vi "均值滤波.vi"(10 "滤波器大小":i32, 11 "inputArray":dbl[][](array[numeric])) -> (1 "中值滤波":dbl[][](array[numeric]), 3 "均值滤波":dbl[][](array[numeric]))   [LabVIEW 2016]
uses:
  <vilib>/Analysis/NI_AALBase.lvlib
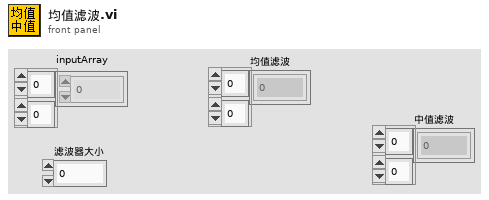
[diagram p1: front panel]
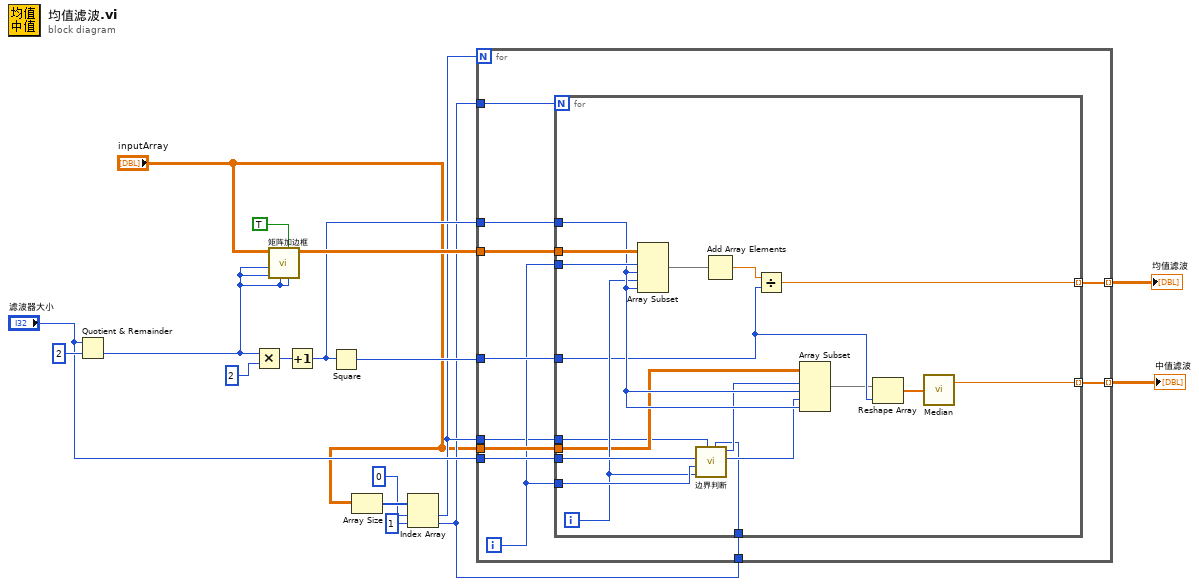
[diagram p0: block diagram]
diagram:
  n1 = Quotient & Remainder(x="滤波器大小", y=2) -> (floor(x/y)=w14:i32)  [unwired: 1 out]
  n2 = Multiply(x=w14, y=2) -> (x*y=w12:i32)
  n3 = call "矩阵加边框.vi"("下边框宽度"=w14, "复制面阵边缘作为边框值"=TRUE, "上边框宽度"=w14, "右边框宽度"=w14, "左边框宽度"=w14, "原面阵"="inputArray") -> ("加边框面阵"=w16:dbl[][])  [unwired: 5 in]
  n4 = Increment(x=w12) -> (x+1=w9:i32)
  n5 = Square(x=w9) -> (x^2=w11:i32)
  n6 = Array Size(array="inputArray") -> (size(s)=w7:i32[])
  n7 = Index Array(array=w7, index #1=0 ("index"), index #2=1 ("index")) -> (element #1=w4:i32, element #2=w3:i32)
  n8 = for {
    N: w4 -> [_]
    tunnel: w16 -> [w28]
    tunnel: w11 -> [w27]
    tunnel: [w26] -> w10 mode=indexing
    tunnel: w9 -> [w25]
    tunnel: "inputArray" -> [w24]
    tunnel: "滤波器大小" -> [w23]
    tunnel: [w21] -> w1 mode=indexing
    tunnel: w4 -> [w20]
    tunnel: w3 -> [w19]
    tunnel: w3 -> [w18]
    i -> [w22]
    n9 = for {
      N: w18 -> [_]
      tunnel: w28 -> [w46]
      tunnel: w22 -> [w45]
      tunnel: w27 -> [w36]
      tunnel: [w43] -> w26 mode=indexing
      tunnel: w25 -> [w41]
      tunnel: w24 -> [w37]
      tunnel: w23 -> [w40]
      tunnel: w22 -> [w39]
      tunnel: [w35] -> w21 mode=indexing
      tunnel: w20 -> [w30]
      tunnel: w19 -> [w29]
      i -> [w38]
      n10 = Array Subset(array=w46, index (row)=w45, length (row)=w41, index (col)=w38, length (col)=w41) -> (w42:dbl[][])
      n11 = call "边界判断.vi"("列"=w29, "行"=w30, "列索引"=w38, "行索引"=w39, "滤波器大小"=w40) -> ("输出列索引"=w33:i32, "输出行索引"=w34:i32)  [unwired: 5 in]
      n12 = Add Array Elements(numeric array=w42) -> (sum=w44:dbl)
      n13 = Divide(x=w44, y=w36) -> (x/y=w43:dbl)
      n14 = Array Subset(array=w37, index (row)=w34, length (row)=w41, index (col)=w33, length (col)=w41) -> (w32:dbl[][])
      n15 = Reshape Array(w32, w36) -> (w31:dbl[])
      n16 = call <vilib>:"Median.vi"("X"=w31) -> ("median"=w35:dbl)  [unwired: 1 out]
    }
  }
  "均值滤波" <- w10
  "中值滤波" <- w1
